vi "Connection Handler.vi"(9 "Error Return":refnum<queue>, 10 "Return Queue":refnum<queue>, 11 "Network Sink Endpoint in":refnum<class "Network Sink Endpoint.lvclass">) -> ()   [LabVIEW 2019, in "Network Sink.lvlib" / "Network Sink Endpoint.lvclass"]
uses:
  <vilib>/gpm_packages/@cs/event-logger/Source/Network Sink/Network Sink Endpoint/Network Sink Endpoint.lvclass
  <vilib>/gpm_packages/@cs/event-logger/Source/Network Sink/Network Sink Endpoint/Network Sink Endpoint.lvclass/Network Sink Endpoint.ctl
  <vilib>/gpm_packages/@cs/Network-Sink/Source/Network Interface/Network Interface/Network Interface.lvclass
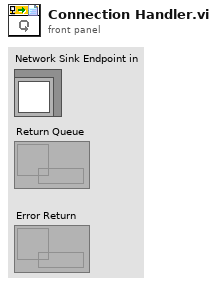
[diagram p1: front panel]
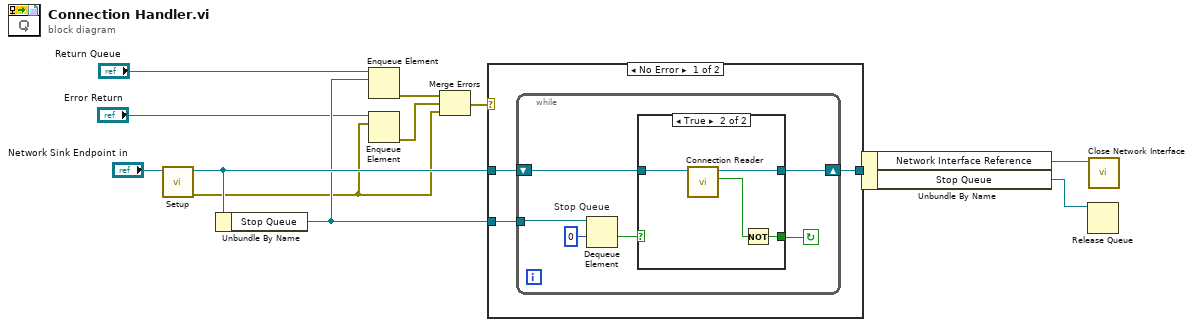
[diagram p0: block diagram]
diagram:
  n1 = call <vilib>:"Setup.vi"("Network Sink Endpoint in"="Network Sink Endpoint in") -> ("error out"=w1:errorcluster, "Network Sink Endpoint out"=w11:refnum<class "Network Sink Endpoint.lvclass">)  [unwired: 9 in]
  n2 = Unbundle By Name(w11) -> ("Stop Queue"=w6:refnum<queue>)
  n3 = Enqueue Element(queue="Return Queue", element=w6) -> (error out=w5:errorcluster)  [unwired: 2 in, 2 out]
  n4 = Enqueue Element(queue="Error Return", element=w1) -> (error out=w2:errorcluster)  [unwired: 2 in, 2 out]
  n5 = Merge Errors(w5, w2, w1) -> (w3:errorcluster)
  n6 = case shown="No Error" w3 {
    tunnel: w11 -> [w15 w28]
    tunnel: [w14 w28] -> w10
    tunnel: w6 -> [w13 _]
    frame No Error {
      n7 = while {
        shift-right: [w18] -> w14
        shift-left: w15 -> [w19]
        tunnel: w13 -> [w21]
        stop <- w16 continue-if-true
        n8 = Dequeue Element "Stop Queue"(queue=w21, timeout in ms (-1)=0) -> (timed out?=w17:bool)  [unwired: 1 in, 3 out]
        n9 = case shown="True" w17 {
          selector: w17 -> [w22 _]
          tunnel: w19 -> [w23 w27]
          tunnel: [w23 w26] -> w18
          tunnel: [w22 w24] -> w16
          frame False {
          }
          frame True {
            n10 = call <vilib>:"Connection Reader.vi"("Network Sink Endpoint in"=w27) -> ("Stop?"=w25:bool, "Network Sink Endpoint out"=w26:refnum<class "Network Sink Endpoint.lvclass">)  [unwired: 8 in, 1 out]
            n11 = Not(x=w25) -> (.not. x?=w24:bool)
          }
        }
      }
    }
    frame Error {
    }
  }
  n12 = Unbundle By Name(w10) -> ("Network Interface Reference"=w9:refnum<data-value>, "Stop Queue"=w8:refnum<queue>)
  n13 = Release Queue(queue=w8) -> ()  [unwired: 2 in, 3 out]
  n14 = call <vilib>:"Close Network Interface.vi"("Network Interface"=w9) -> ()  [unwired: 10 in, 1 out]
